vi "ConfigureTrig.vi"(8 "error in (no error)":errorcluster, 11 "reference in":refnum<class "niMmWave_Transceiver.lvclass">) -> (0 "error out":errorcluster, 3 "reference out":refnum<class "niMmWave_Transceiver.lvclass">)   [LabVIEW 2019, in "niMmWave_Transceiver.lvclass"]
uses:
  niMmWave_Transceiver.lvclass
  C:/Barkhausen mmWave radar/Development/modules/mmw_instrument/src_LabVIEW/Host/SubVIs/mmWave instrument_class/mmWave instrument.lvclass
  FPGA/SubVIs/Utility/FPGA driver trigger destination.ctl
  FPGA/SubVIs/Utility/FPGA driver trigger source.ctl
  mmWave instrument_class/mmWave instrument.lvclass
  FPGA/SubVIs/Utility/FPGA Utility.lvlib
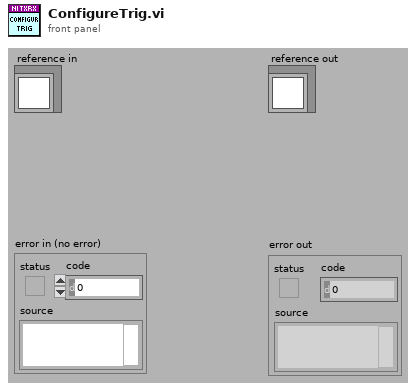
[diagram p1: front panel]
types:
  T1 = typedef "FPGA Utility.lvlib/FPGA driver trigger source.ctl" = enum16{"Use Tclk", "PXI_Trig", "Aurora RX trig"}
  T2 = typedef "FPGA Utility.lvlib/FPGA driver trigger destination.ctl" = enum16{"None", "Source trig", "Synced trig", "Delayed sync"}
  T3 = typedef "niMmWave_Transceiver.lvclass/ObjectAttributesRef.ctl" = refnum<data-value>
  T4 = typedef "mmWave instrument.lvclass/ObjectAttributes.ctl" = cluster{"mode":T5, "instr state":T6, "Max Fs":dbl, "Equalization coeff":cdb[], "LO sync en":bool, "Trig sync en":bool, "LO sources":T7, "LO Export":T8, "Fc.range":cluster{"min":dbl, "max":dbl}, "Sync mode":T9, "equalization en":bool, "sequence":string[]}
  T5 = typedef "mmWave instrument.lvclass/Instrument mode.ctl" = enum16{"RF", "IF", "BB"}
  T6 = typedef "mmWave instrument.lvclass/Instrument state.ctl" = enum16{"Off", "Initialization", "Configuration", "Running", "Calibration"}
  T7 = typedef "mmWave HW Control.lvlib/LO sources.ctl" = cluster{"RX/LO1 src":string, "TX/LO1 src":string, "LO2 src":string}
  T8 = typedef "mmWave HW Control.lvlib/LO export.ctl" = cluster{"TX LO1 export":bool, "TX LO1 export level":dbl, "RX LO1 export":bool, "RX LO1 export level":dbl, "LO2 export":bool, "LO2 export level":dbl}
  T9 = typedef "mmWave instrument.lvclass/Sync mode.ctl" = enum16{"Slave", "Master"}
  T10 = typedef "niMmWave_Transceiver.lvclass/ObjectAttributes.ctl" = cluster{"session":T11[], "HW.RX resources":T25, "RF config":T26, "RX trigger options":T27, "TX trigger options":T27, "RX samples":i32, "Downloaded Bursts":map{string, T28}, "TX Fs":dbl, "RX Fs":dbl, "burst sequence":string[]}
  T11 = typedef "Session.ctl" = cluster{"3620 session":refnum<queue>, "tx baseband session":T12, "rx baseband session":T20, "tx gain (dB)":dbl, "rx gain (dB)":dbl, "hardware configuration":T21, "gain ranging":T23[], "pxi trigger bus information":T24}
  T12 = typedef "Tx Baseband Session.ctl" = cluster{"3610 session":T13, "7902 reference":T19}
  T13 = typedef "ni3610_and_ni3630_Driver_Lib.lvlib/Main Settings.ctl" = cluster{"VISA resource name":refnum<visa-resource-name>, "Address Space":T14, "window_offset":u32, "register_addresses":T15, "required_MM_fpga_version":cluster{"signature":u32, "hardware":u32, "current revision":u32, "oldest revision":u32}, "CPLD Oldest Compat Version ":cluster{"hardware":u32, "CPLD firmware":u32}, "MM_FPGA_image_location":string, "is_init":bool, "card_type":T16, "DacLmkConfigFileName":string, "AdcLmkConfigFileName":string, "AdcConfigFileName":string, "DacConfigFileName_RevA":string, "DacConfigFileName_RevB":string, "Mulde hardware revision":u8, "bypass DAC PLL\n":bool, "IQ Card Revision":T17, "board capability":T18}
  T14 = typedef "VISA Register Access Address Space.ctl" = u16
  T15 = typedef "ni3610_and_ni3630_Driver_Lib.lvlib/Register Adresses.ctl" = cluster{"MM based Registers":cluster{"Revision":u32, "OldestCompatRev":u32, "signature":u32, "scratch":u32, "LedControl":u32, "BoardHwRev":u32, "BoardControl":u32, "ThermalStatus":u32, "BasebandStatus":u32, "BasebandControl":u32, "BasebandAuxSetup":u32, "BasebandAuxStatus":u32, "LmkSyncOutSetup":u32, " AdcSyncOutSetup":u32, " InjSyncOutSetup":u32, " PxiTrig0OutSetup":u32, " PxiTrig1OutSetup":u32, " PxiTrig2OutSetup":u32, " PxiTrig3OutSetup":u32, " PxiTrig4OutSetup":u32, " PxiTrig5OutSetup":u32, " PxiTrig6OutSetup":u32, " PxiTrig7OutSetup":u32}, "CPLD based Registers":cluster{"SlaveSignature":u32, "SlaveRevision":u32, "SlaveOldestCompatRev":u32, "SlaveScratch":u32, "SlaveSetup":u32, "SlaveStatus":u32, "IDacReg_offset":u32, "LMKRegGrp0_offset":u32, "QDacReg_offset":u32, "BrdTempSensorVal":u32, "TempSensorPowerDown":u32, "GPIOReg_offset":u32, "IAdcReg_offset":u32, "QAdcReg_offset":u32, "LMKRegGrp1_offset":u32, "QadcTempSensorVal":u32, "IadcTempSensorVal":u32, "RevisionReg":u32, "VcxoReg":u32, "CpldStatusReg":u32, "PowerReg":u32, "VBiasEnReg":u32, "ExtRefOeReg":u32, "QdacCtrlReg":u32, "QdacStatusReg":u32, "IdacCtrlReg":u32, "IdacStatusReg":u32, "QdacJtagIn":u32, "QdacJtagOut":u32, "IdacJtagIn":u32, "IdacJtagOut":u32, "IqDcSetupReg":u32, "QadcStatusReg":u32, "IadcStatusReg":u32, "BrdSetupReg":u32, "IqDcRevisionReg":u32, "PllStatusReg":u32, "EndpointScratchReg":u32, "AdcSyncCfgReg":u32, "IqCardOpampReg":u32}, "CPLD Register Offset":u32, "MM  Register Offset":u32, " PxiTrig0OutSetup":u32}
  T16 = typedef "ni3610_and_ni3630_Driver_Lib.lvlib/Base Card Type.ctl" = enum16{"unspecified", "ADC", "DAC"}
  T17 = typedef "ni3610_and_ni3630_Driver_Lib.lvlib/IQ Card Revision.ctl" = enum16{"RevA", "RevB", "RevC", "RevD"}
  T18 = typedef "ni3610_and_ni3630_Driver_Lib.lvlib/Board Capability.ctl" = cluster{"baseband sync":enum16{"no baseband sync", "baseband sync"}}
  T19 = typedef "Blank FPGA Reference.ctl" = refnum<k20>
  T20 = typedef "Rx Baseband Session.ctl" = cluster{"3630 session":T13, "7902 reference":T19}
  T21 = typedef "Hardware Configuration.ctl" = cluster{"direction":T22, "baseband only":bool}
  T22 = typedef "Direction.ctl" = enum16{"Transceiver", "Receiver", "Transmitter"}
  T23 = typedef "Gain Ranging.ctl" = cluster{"gain ranging active scope":string, "gain ranging stream session":refnum<k20>}
  T24 = typedef "PXI Trigger Bus Info.ctl" = cluster{"chassis resource name":refnum<visa-resource-name>, "7902R (TX)":i16, "3610 (TX)":i16, "3620 (IF)":i16, "3630 (RX)":i16, "7902R (RX)":i16}
  T25 = typedef "mmWave HW Control.lvlib/HW TXRX resources cluster.ctl" = cluster{"TX_DAC":refnum<visa-resource-name>, "TX_FPGA":tag, "IF":tag, "RX_ADC":refnum<visa-resource-name>, "RX_FPGA":tag}
  T26 = typedef "mmWave HW Control.lvlib/HW TXRX RF config cluster.ctl" = cluster{"TX.Frequency":dbl, "TX.Gain":dbl, "TX.mmWave adapter":string, "RX.Frequency":dbl, "RX.Gain":dbl, "RX.mmWave adapter":string}
  T27 = typedef "TX trigger config.ctl" = cluster{"delay":dbl, "trig source":T1, "PXI src":i32, "export":T2, "PXI dest":i32}
  T28 = typedef "niMmWave_Transceiver.lvclass/BurstInfo.ctl" = cluster{"starting addr":u32, "end addr":u32}
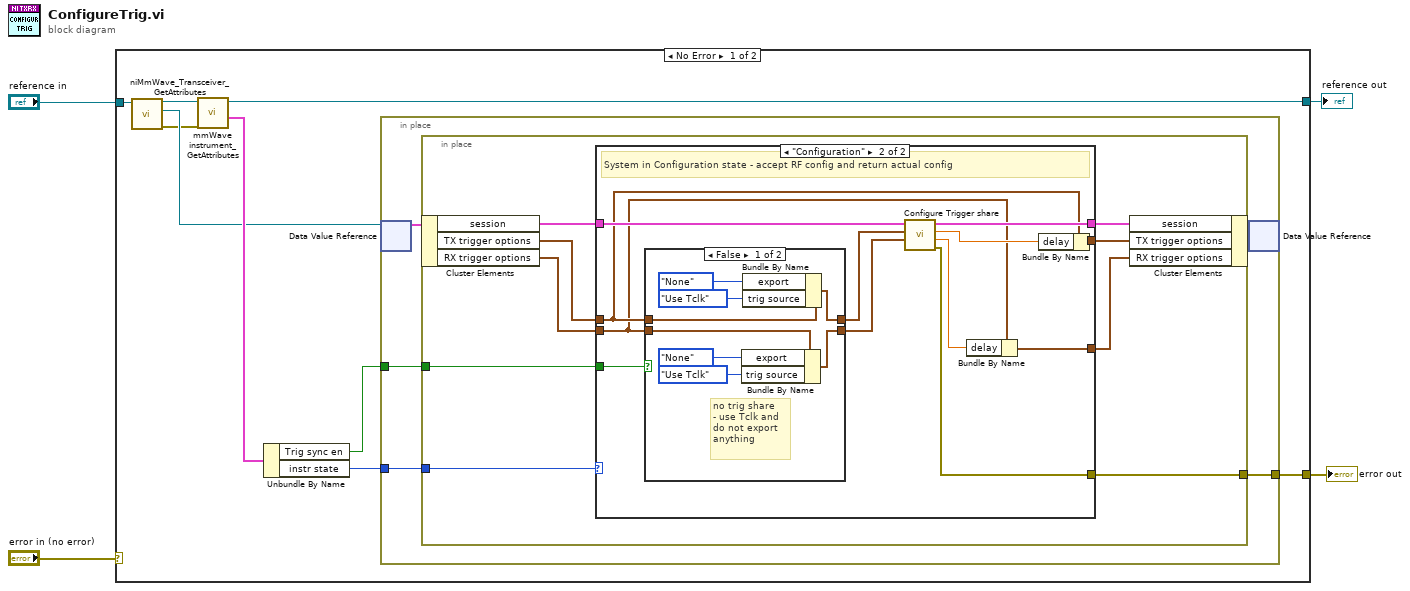
[diagram p0: block diagram]
diagram:
  n1 = case shown="No Error" "error in (no error)" {
    selector: "error in (no error)" -> [_ w54]
    tunnel: [w6 w54] -> w3
    tunnel: [w11 w53] -> w1
    tunnel: "reference in" -> [w12 w53]
    frame No Error {
      n2 = call "niMmWave_Transceiver_GetAttributes.vi"("reference in"=w12) -> ("error out"=w8:errorcluster, "attributes ref"=w9:T3, "reference out"=w13:refnum<class "niMmWave_Transceiver.lvclass">)  [unwired: 7 in, 1 out]
      n3 = call "mmWave instrument_GetAttributes.vi"("error in (no error)"=w8, "reference in"=w13) -> ("attributes"=w10:T4, "reference out"=w11:refnum<class "niMmWave_Transceiver.lvclass">)  [unwired: 6 in, 2 out]
      n4 = Unbundle By Name(w10) -> ("Trig sync en"=w5:bool, "instr state"=w7:T6)
      n5 = in-place {
        in-place-border: w7 -> [w16]
        in-place-border: [w15] -> w6
        in-place-border: w5 -> [w14]
        n6 = in-place-dvr #1(w9) -> (w18:T10)  [unwired: 1 out]
        n7 = in-place {
          in-place-border: w16 -> [w25]
          in-place-border: [w22] -> w15
          in-place-border: w14 -> [w19]
          n8 = in-place-cluster #2(w18) -> ("session"=w27:T11[], "TX trigger options"=w24:T27, "RX trigger options"=w23:T27)
          n9 = case shown="\"Configuration\"" w25 {
            tunnel: w27 -> [w30 w42]
            tunnel: [w30 w41] -> w26
            tunnel: w24 -> [w29 w33]
            tunnel: w23 -> [w28 w31]
            tunnel: [_ w40] -> w22
            tunnel: [w29 w39] -> w20
            tunnel: [w28 w38] -> w21
            tunnel: w19 -> [_ w35]
            frame "Off", Default {
            }
            frame "Configuration" {
              # "System in Configuration state - accept RF config and return actual config"
              n10 = case shown="False" w35 {
                tunnel: [w49 w52] -> w34
                tunnel: w33 -> [w50 w52]
                tunnel: [w44 w51] -> w32
                tunnel: w31 -> [w43 w51]
                frame False {
                  # "no trig share\n- use Tclk and \ndo not export \nanything"
                  n11 = Bundle By Name(cluster=w43, "export"=FPGA_driver_trigger_destination."None", "trig source"=FPGA_driver_trigger_source."Use Tclk") -> (w44:T27)
                  n12 = Bundle By Name(cluster=w50, "export"=FPGA_driver_trigger_destination."None", "trig source"=FPGA_driver_trigger_source."Use Tclk") -> (w49:T27)
                }
                frame True {
                  # "trig share\nenables\nuse settings\nfrom ini"
                }
              }
              n13 = call "Configure Trigger share.vi"("RX trigger options"=w32, "TX trigger options"=w34, "session in"=w42) -> ("error out"=w40:errorcluster, "actual rx delay"=w36:dbl, "actual tx delay"=w37:dbl, "session out"=w41:T11[])  [unwired: 5 in]
              n14 = Bundle By Name(cluster=w31, "delay"=w36) -> (w38:T27)
              n15 = Bundle By Name(cluster=w33, "delay"=w37) -> (w39:T27)
            }
          }
          n16 = in-place-cluster #2("session"=w26, "TX trigger options"=w20, "RX trigger options"=w21) -> (w17:T10)
        }
        n17 = in-place-dvr #1(w17) -> ()  [unwired: 2 out]
      }
    }
    frame Error {
    }
  }
  "error out" <- w3
  "reference out" <- w1
